vi "Handle Error.vi"(8 "error in (no error)":errorcluster, 11 "CI Mediator in":refnum<class "CI Mediator.lvclass">) -> (0 "error out":errorcluster, 2 "stop actor?":bool=TRUE, 3 "CI Mediator out":refnum<class "CI Mediator.lvclass">)   [LabVIEW 2014, in "CI Mediator.lvlib" / "CI Mediator.lvclass"]
doc: "(<B>Filename</B>: Actor Framework.lvlib:Actor.lvclass:Handle Error.vi)\n\nDefines how the actor handles an error that occurred while processing a message. By default, this method does nothing except stop the actor."
uses:
  CI Mediator.lvclass
  <vilib>/ActorFramework/Actor/Actor.lvclass
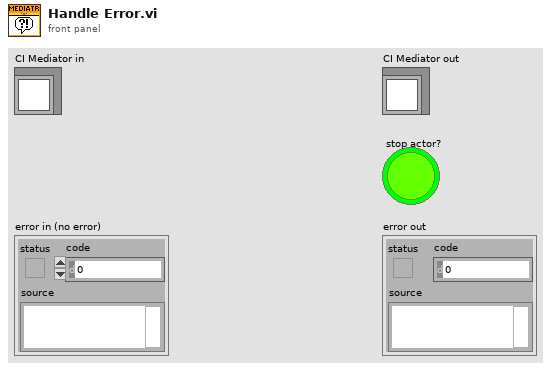
[diagram p1: front panel]
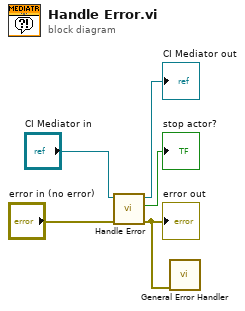
[diagram p0: block diagram]
diagram:
  n1 = call-parent "Handle Error.vi"("error in (no error)"="error in (no error)", "Actor in"="CI Mediator in") -> ("error out"=w1:errorcluster, "stop actor?"=→"stop actor?":bool, "Actor out"=→"CI Mediator out":refnum<class "CI Mediator.lvclass">)  [unwired: 7 in]
  "error out" <- w1
  n2 = call <vilib>:"General Error Handler.vi"("error in (no error)"=w1) -> ()  [unwired: 10 in, 5 out]
